vi "Global_Shifter_SM_Data Out.vi"() -> ()   [LabVIEW 2016]
panel:
  out "High Gear Enabled":bool
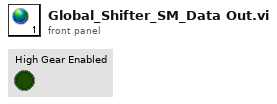
[diagram p1: front panel]
diagram:
